vi "operacja.vi"(4 "amplituda in":T4=10.0 caption="Frequency", 5 "z jakim?":T2 items=["sin", "square", "sawtooth", "noise"], 6 "czestotl [Hz]":T5 caption="Frequency", 7 "dzialanie":T3 items=["+", "-", "*", "/", ""], 8 "millisecond timer value":u32, 11 "jaki sygna³?":T1 items=["sin", "square", "sawtooth", "noise"]) -> (1 "Array":T4[](array[typedef]), 2 "amplituda out":T4 caption="Frequency", 3 "x pocz out":T6)   [LabVIEW 2016]
uses:
  lab4/genetrator/Control 2.ctl
  lab4/genetrator/Control 3.ctl
  lab4/genetrator/Control 1.ctl
  lab4/genetrator/Control 6.ctl
  lab4/genetrator/Control 5.ctl
  lab4/genetrator/Control 4.ctl
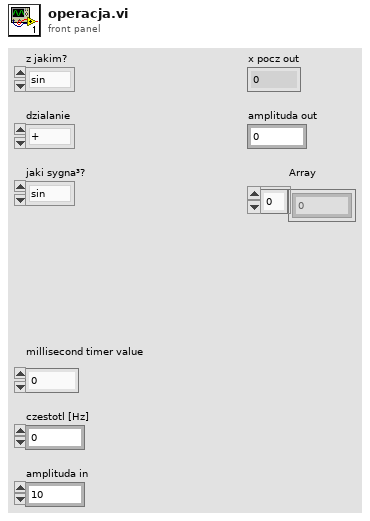
[diagram p1: front panel]
types:
  T1 = typedef "Control 4.ctl" = u16
  T2 = typedef "Control 5.ctl" = u16
  T3 = typedef "Control 6.ctl" = u16
  T4 = typedef "Control 2.ctl" = dbl
  T5 = typedef "Control 1.ctl" = dbl
  T6 = typedef "Control 3.ctl" = dbl
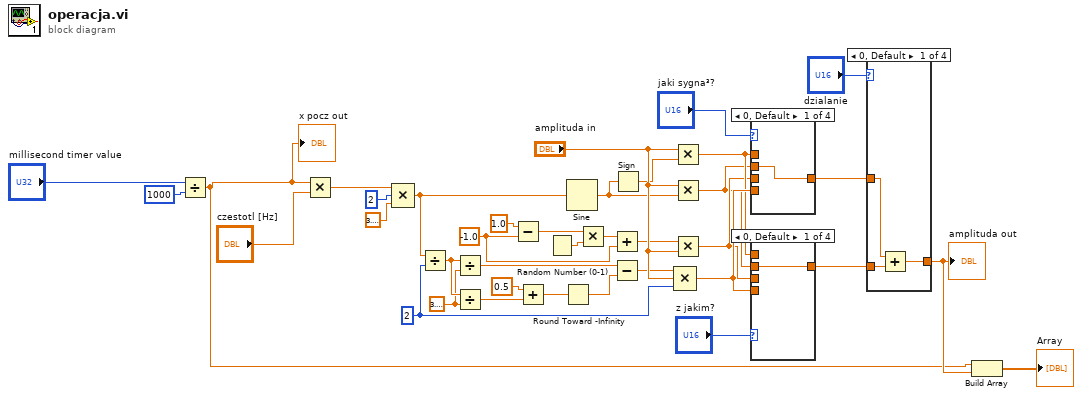
[diagram p0: block diagram]
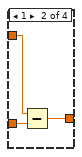
[diagram p2: hidden frame]
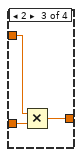
[diagram p3: hidden frame]
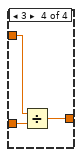
[diagram p4: hidden frame]
diagram:
  w32 = 2
  w19 = 3.141592653589793
  w7 = -1.0 ("x")
  n1 = Divide(x="millisecond timer value", y=1000) -> (x/y=w27:dbl)
  "x pocz out" <- w27
  n2 = Multiply(x=w27, y="czestotl [Hz]") -> (x*y=w29:T5)
  n3 = Compound Arithmetic op=MULTIPLY(w29, 2, 3.141592653589793) -> (w30:T5)
  n4 = Divide(x=w30, y=w32) -> (x/y=w31:T5)
  n5 = Divide(x=w31, y=w19) -> (x/y=w20:T5)
  n6 = Divide(x=w31, y=w19) -> (x/y=w23:T5)
  n7 = Subtract(x=1.0, y=w7) -> (x-y=w9:dbl)
  n8 = Add(x=0.5, y=w23) -> (x+y=w22:T5)
  n9 = Random Number (0-1)() -> (number: 0 to 1=w10:dbl)
  n10 = Round Toward -Infinity(1:w22) -> (0:w21:T5)
  n11 = Sine(x=w30) -> (sin(x)=w15:T5)
  n12 = Multiply(x=w9, y=w10) -> (x*y=w11:dbl)
  n13 = Add(x=w11, y=w7) -> (x+y=w12:dbl)
  n14 = Subtract(x=w20, y=w21) -> (x-y=w24:T5)
  n15 = Sign(1:w15) -> (0:w16:T5)
  n16 = Multiply(x="amplituda in", y=w16) -> (x*y=w17:T4)
  n17 = Multiply(x="amplituda in", y=w15) -> (x*y=w13:T4)
  n18 = Multiply(x=w12, y="amplituda in") -> (x*y=w14:T4)
  n19 = Compound Arithmetic op=MULTIPLY(w24, "amplituda in", w32) -> (w25:T5)
  n20 = case shown="0, Default" "jaki sygna³?" {
    tunnel: w13 -> [w38 _ _ _]
    tunnel: w17 -> [_ w39 _ _]
    tunnel: w25 -> [_ _ w40 _]
    tunnel: w14 -> [_ _ _ w41]
    tunnel: [w38 w39 w40 w41] -> w2
    frame 0, Default {
    }
    frame 1 {
    }
    frame 2 {
    }
    frame 3 {
    }
  }
  n21 = case shown="0, Default" "z jakim?" {
    tunnel: w13 -> [w42 _ _ _]
    tunnel: w17 -> [_ w43 _ _]
    tunnel: w25 -> [_ _ w44 _]
    tunnel: w14 -> [_ _ _ w45]
    tunnel: [w42 w43 w44 w45] -> w3
    frame 0, Default {
    }
    frame 1 {
    }
    frame 2 {
    }
    frame 3 {
    }
  }
  n22 = case shown="0, Default" "dzialanie" {
    tunnel: w2 -> [w48 w51 w54 w57]
    tunnel: w3 -> [w47 w50 w53 w56]
    tunnel: [w46 w49 w52 w55] -> w37
    frame 0, Default {
      n23 = Add(x=w48, y=w47) -> (x+y=w46:T4)
    }
    frame 1 {
      n24 = Subtract(x=w51, y=w50) -> (x-y=w49:T4)
    }
    frame 2 {
      n25 = Multiply(x=w54, y=w53) -> (x*y=w52:T4)
    }
    frame 3 {
      n26 = Divide(x=w57, y=w56) -> (x/y=w55:T4)
    }
  }
  "amplituda out" <- w37
  n27 = Build Array(w27, w37) -> (→"Array":T4[])
